vi "AdvancedConfig.vi"(8 "error in":errorcluster {"code" format="Error %.0f"}, 11 "MainFGV_data":T3={"TestDir"=path "", "TestName"="", "task"="", "data_file"=refnum, "AcqQueue"=refnum, "StartTime"=timestamp(0 s since 1904-01-01), "config_channels"=[], "DAQmx Device"="", "Advanced"={"rate"=1652.0, "duration"=1.0, "thr"=100.0, "preTrigger"=100.0, "cutoff"=-3.0, "Filtro"=enum."Desativado", "highPass"=1000.0, "lowPass"=1000.0, "updateTime"=50.0}, "running"=FALSE, "hammerIndex"=0, "session"="localhost"} {"Advanced"."updateTime" format="%#_g ms"; "Advanced"."lowPass" format="%#_g Hz"; "Advanced"."highPass" format="%#_g Hz"; "Advanced"."cutoff" format="%#_g dB"; "Advanced"."preTrigger" format="%#_g ms"; "Advanced"."thr" format="%#_g N"; "Advanced"."duration" format="%#_g s"; "Advanced"."rate" min=1652.0 max=51200.0 format="%#_g Hz"}) -> (0 "error out":errorcluster {"code" format="Error %.0f"}, 3 "MainFGV_data out":T3={"TestDir"=path "", "TestName"="", "task"="", "data_file"=refnum, "AcqQueue"=refnum, "StartTime"=timestamp(0 s since 1904-01-01), "config_channels"=[], "DAQmx Device"="", "Advanced"={"rate"=1652.0, "duration"=1.0, "thr"=100.0, "preTrigger"=100.0, "cutoff"=-3.0, "Filtro"=enum."Desativado", "highPass"=1000.0, "lowPass"=1000.0, "updateTime"=50.0}, "running"=FALSE, "hammerIndex"=0, "session"="localhost"} {"Advanced"."updateTime" format="%#_g ms"; "Advanced"."lowPass" format="%#_g Hz"; "Advanced"."highPass" format="%#_g Hz"; "Advanced"."cutoff" format="%#_g dB"; "Advanced"."preTrigger" format="%#_g ms"; "Advanced"."thr" format="%#_g N"; "Advanced"."duration" format="%#_g s"; "Advanced"."rate" min=1652.0 max=51200.0 format="%#_g Hz"})   [LabVIEW 2018]
uses:
  Processing/processing_mods.ctl
  MainFGV_data.ctl
  config_board.ctl
  AdvancedConfig.ctl
  NI9234_AcqRates.ctl
panel:
  in  "updateTime":dbl=50.0 caption="Intervalo de atualização" min=1.0 max=1000.0 format="%#_g ms"
  in  "rate":T1=enum."2048 Hz" caption="Taxa de aquisição"
  in  "lowPass":dbl=1000.0 caption="Passa baixa" format="%#_g Hz"
  in  "highPass":dbl=1.0 caption="Passa alta" format="%#_g Hz"
  in  "Filtro":T2(ring)=enum."Passa alta"
  in  "cutoff":dbl=-6.0 caption="Cutoff amplitude [dB]" max=-0.01 format="%#_g dB"
  in  "preTrigger":dbl=100.0 caption="Pre-trigger" min=0.0 max=60000.0 format="%#_g ms"
  in  "thr":dbl=10.0 caption="Limiar de força" min=1.0 format="%#_g N"
  in  "duration":dbl=1.0 caption="Duração" min=0.001 max=60.0 format="%#_g s"
  in  "cancel":bool
  in  "ok":bool
  # "Configurações avançadas"
  # "Detecção da batida"
  # "Apresentação do resultado"
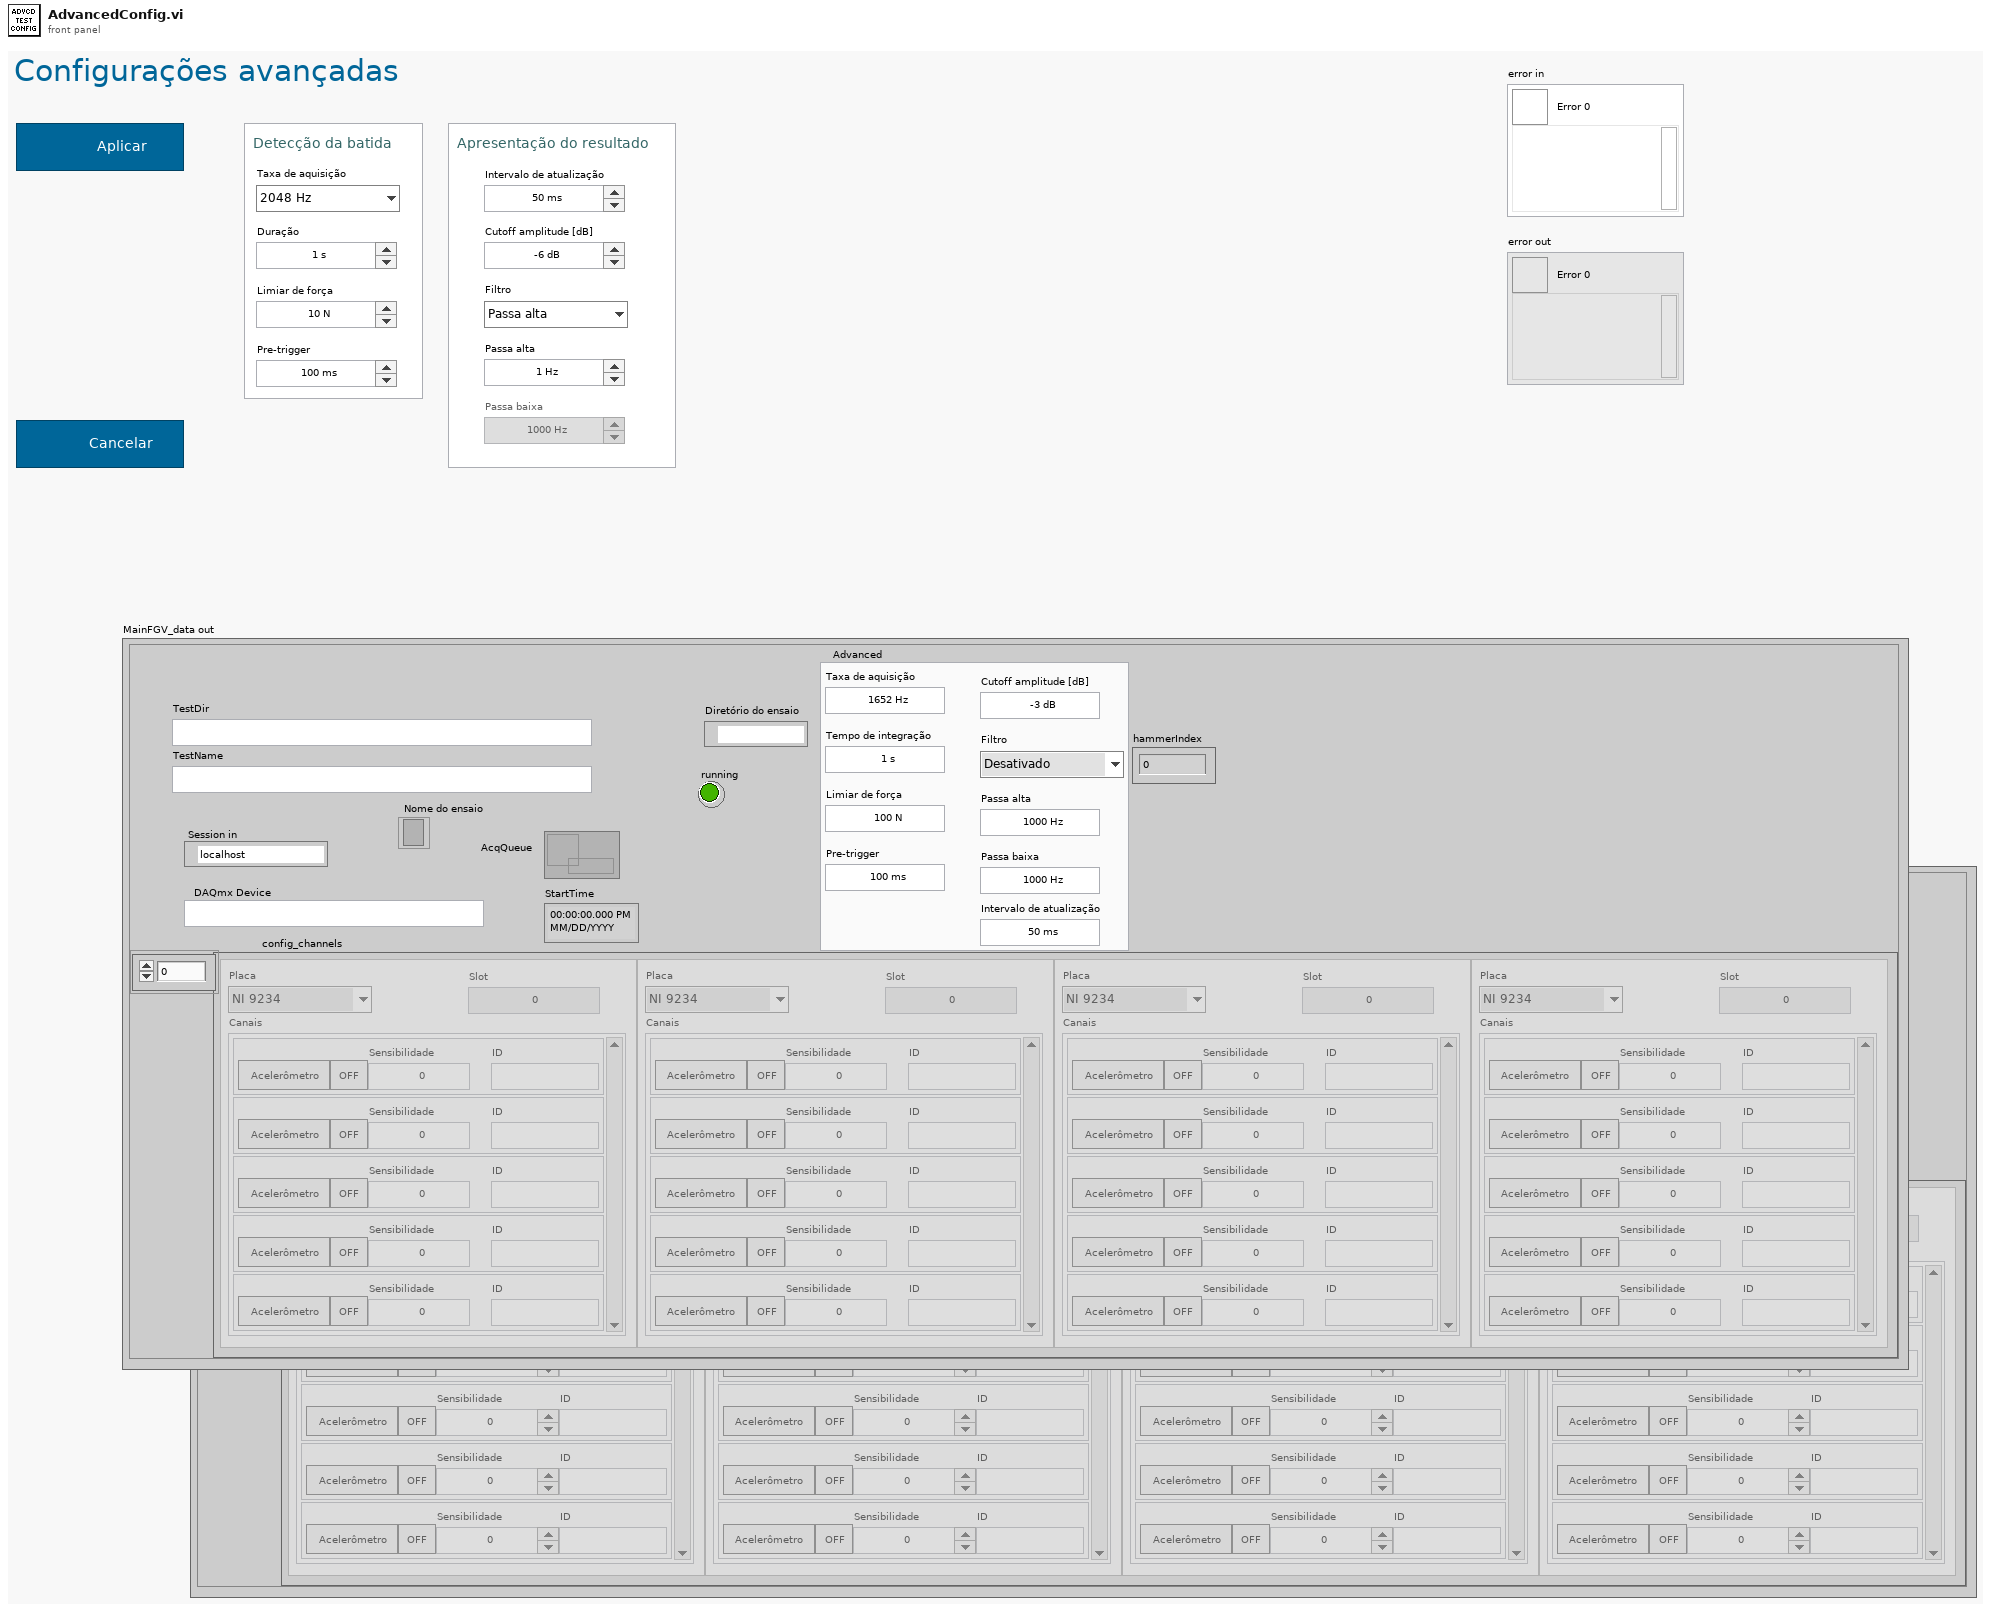
[diagram p1: front panel]
types:
  T1 = typedef "NI9234_AcqRates.ctl" = enum16{"51200 Hz", "25600 Hz", "17066 Hz", "12800 Hz", "10240 Hz", "8533 Hz", "7314 Hz", "6400 Hz", "5689 Hz", "5120 Hz", "4654 Hz", "4267 Hz", "3938 Hz", "3657 Hz", "3413 Hz", "3200 Hz", "3012 Hz", "2844 Hz", "2694 Hz", "2560 Hz", "2438 Hz", "2327 Hz", "2226 Hz", "2133 Hz", "2048 Hz", "1969 Hz", "1896 Hz", "1828 Hz", "1765 Hz", "1706 Hz", "1651 Hz"}
  T2 = enum16{"Desativado", "Passa banda", "Passa alta", "Passa baixa"}
  T3 = typedef "MainFGV_data.ctl" = cluster{"TestDir":path, "TestName":string, "task":refnum<k21>, "data_file":refnum<file>, "AcqQueue":refnum<queue>, "StartTime":timestamp, "config_channels":T4[], "DAQmx Device":tag, "Advanced":T5, "running":bool, "hammerIndex":i32, "session":refnum<k21>}
  T4 = typedef "config_board.ctl" = cluster{"board":enum16{"NI 9234", "NI 9205", "Não aplicável"}, "channels":cluster{"type":bool, "active":bool, "sens":dbl, "ID":string}[], "Slot":i32}
  T5 = typedef "AdvancedConfig.ctl" = cluster{"rate":dbl, "duration":dbl, "thr":dbl, "preTrigger":dbl, "cutoff":dbl, "Filtro":enum16{"Desativado", "Passa banda", "Passa alta", "Passa baixa"}, "highPass":dbl, "lowPass":dbl, "updateTime":dbl}
  T6 = typedef "processing_mods.ctl" = enum16{"newData", "SetConfig", "setHammer"}
  T7 = enum8{"Enabled", "Disabled", "Disabled and Grayed Out"}
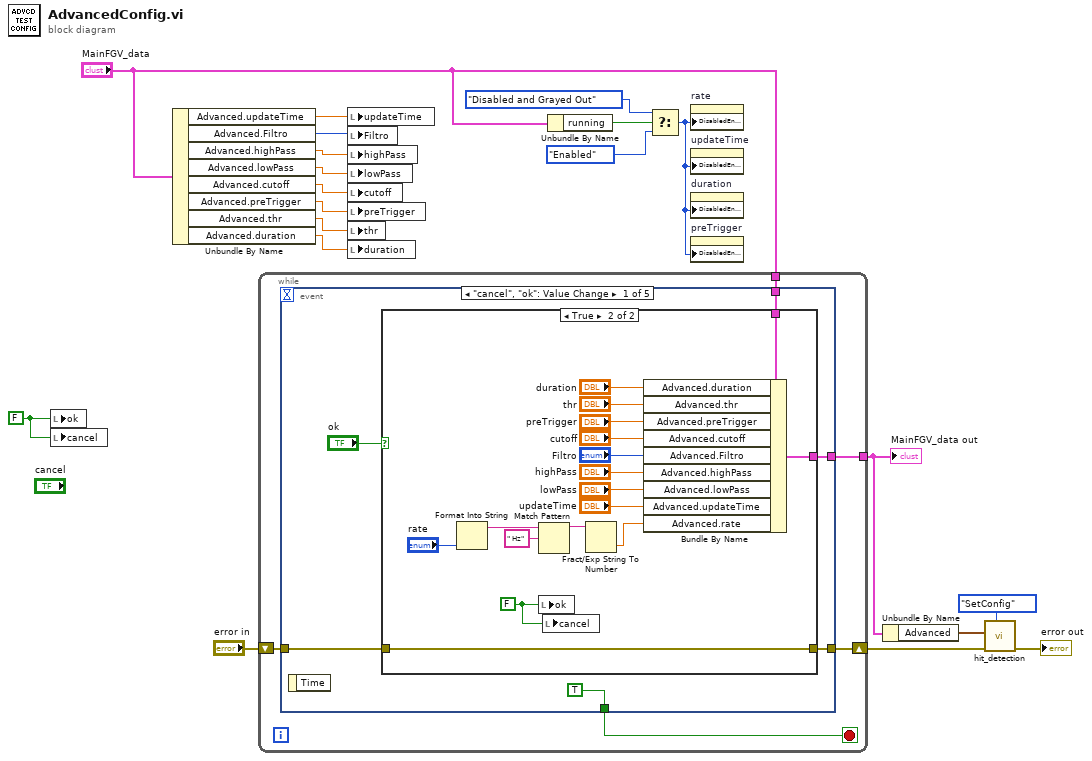
[diagram p0: block diagram]
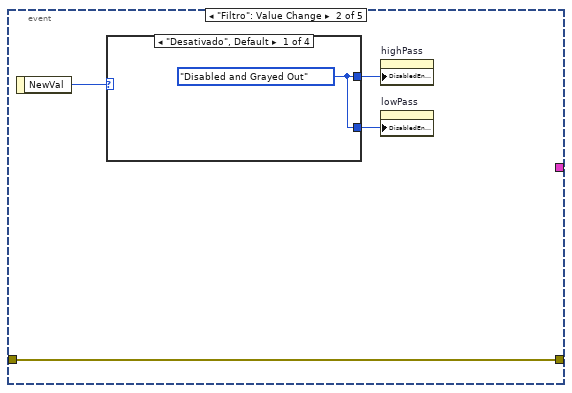
[diagram p3: hidden frame]
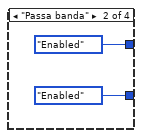
[diagram p4: hidden frame]
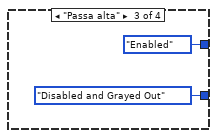
[diagram p5: hidden frame]
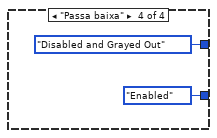
[diagram p6: hidden frame]
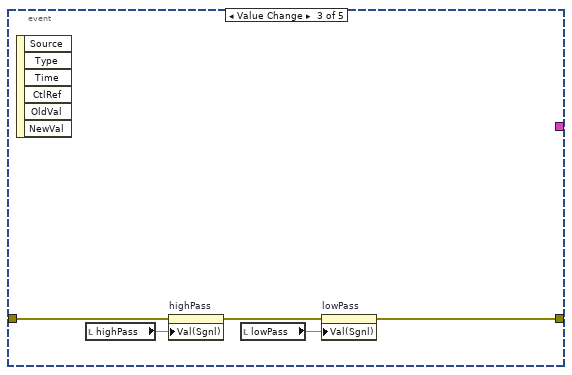
[diagram p7: hidden frame]
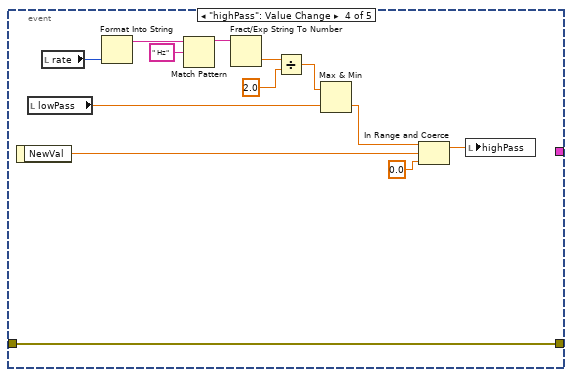
[diagram p8: hidden frame]
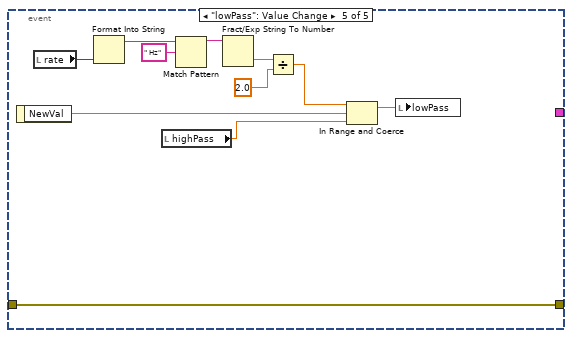
[diagram p9: hidden frame]
diagram:
  w19 = FALSE ("OK")
  n1 = local write "ok"(w19) -> ()
  n2 = local write "cancel"(w19) -> ()
  n3 = Unbundle By Name("MainFGV_data") -> ("Advanced.updateTime"=w8:dbl, "Advanced.Filtro"=w7:T2, "Advanced.highPass"=w6:dbl, "Advanced.lowPass"=w5:dbl, "Advanced.cutoff"=w4:dbl, "Advanced.preTrigger"=w3:dbl, "Advanced.thr"=w2:dbl, "Advanced.duration"=w1:dbl)
  n4 = while {
    shift-right: [w24] -> w14
    shift-left: "error in" -> [w21]
    tunnel: "MainFGV_data" -> [w23]
    tunnel: [w22] -> w13
    stop <- w25 stop-if-true
    n5 = event shown="[0] \"cancel\", \"ok\": Value Change" {
      selector: _ -> [_ _ _ _ _]
      dyn-events: _ -> [_ _ _ _ _]
      timeout: _ -> [_ _ _ _ _]
      tunnel: [TRUE ("OK") _ _ _ _] -> w25
      tunnel: w21 -> [w29 w51 w63 w67 w83]
      tunnel: [w28 w51 w62 w67 w83] -> w24
      tunnel: w23 -> [w31 _ _ _ _]
      tunnel: [w30 _ _ _ _] -> w22
      event "cancel", "ok": Value Change {
        n6 = event-data() -> ()  [unwired: 1 in, 1 out]
        n7 = case shown="True" "ok" {
          tunnel: w31 -> [w33 w50]
          tunnel: [w33 w49] -> w30
          tunnel: w29 -> [w32 w48]
          tunnel: [w32 w48] -> w28
          frame False {
          }
          frame True {
            w47 = FALSE ("OK")
            n8 = Format Into String("rate") -> (resulting string=w37:string)  [unwired: 3 in, 1 out]
            n9 = Match Pattern(string=w37, regular expression=" Hz") -> (before substring=w39:string)  [unwired: 1 in, 3 out]
            n10 = local write "ok"(w47) -> ()
            n11 = local write "cancel"(w47) -> ()
            n12 = Fract/Exp String To Number(string=w39) -> (number=w35:dbl)  [unwired: 3 in, 1 out]
            n13 = Bundle By Name(cluster=w50, "Advanced.duration"="duration", "Advanced.thr"="thr", "Advanced.preTrigger"="preTrigger", "Advanced.cutoff"="cutoff", "Advanced.Filtro"="Filtro", "Advanced.highPass"="highPass", "Advanced.lowPass"="lowPass", "Advanced.updateTime"="updateTime", "Advanced.rate"=w35) -> (w49:T3)
          }
        }
      }
      event "Filtro": Value Change {
        n14 = event-data() -> ("NewVal"=w54:T2)  [unwired: 1 in]
        n15 = case shown="\"Desativado\", Default" w54 {
          tunnel: [w55 T7."Enabled" ("Disabled") T7."Enabled" ("Disabled") T7."Disabled and Grayed Out" ("Disabled")] -> w53
          tunnel: [w55 T7."Enabled" ("Disabled") T7."Disabled and Grayed Out" ("Disabled") T7."Enabled" ("Disabled")] -> w52
          frame "Desativado", Default {
            w55 = T7."Disabled and Grayed Out" ("Disabled")
          }
          frame "Passa banda" {
          }
          frame "Passa alta" {
          }
          frame "Passa baixa" {
          }
        }
        n16 = property on="highPass" class="DigNum (strict)"("DisabledEnum"=w53) -> ()  [unwired: 2 in, 2 out]
        n17 = property on="lowPass" class="DigNum (strict)"("DisabledEnum"=w52) -> ()  [unwired: 2 in, 2 out]
      }
      event Value Change {
        n18 = event-data() -> ()  [unwired: 1 in, 6 out]
        n19 = local read "highPass"() -> (w66:dbl)
        n20 = property on="highPass" class="DigNum (strict)"(error in=w63, "Val(Sgnl)"=w66) -> (error out=w64:errorcluster)  [unwired: 1 in, 1 out]
        n21 = local read "lowPass"() -> (w65:dbl)
        n22 = property on="lowPass" class="DigNum (strict)"(error in=w64, "Val(Sgnl)"=w65) -> (error out=w62:errorcluster)  [unwired: 1 in, 1 out]
      }
      event "highPass": Value Change {
        n23 = event-data() -> ("NewVal"=w79:dbl)  [unwired: 1 in]
        n24 = local read "lowPass"() -> (w69:dbl)
        n25 = local read "rate"() -> (w76:T1)
        n26 = Format Into String(w76) -> (resulting string=w73:string)  [unwired: 3 in, 1 out]
        n27 = Match Pattern(string=w73, regular expression=" Hz") -> (before substring=w75:string)  [unwired: 1 in, 3 out]
        n28 = Fract/Exp String To Number(string=w75) -> (number=w72:dbl)  [unwired: 3 in, 1 out]
        n29 = Divide(x=w72, y=2.0) -> (x/y=w70:dbl)
        n30 = Max & Min(x=w70, y=w69) -> (min(x,y)=w68:dbl)  [unwired: 1 out]
        n31 = In Range and Coerce(upper limit=w68, x=w79, lower limit=0.0) -> (coerced(x)=w77:dbl)  [unwired: 1 out]
        n32 = local write "highPass"(w77) -> ()
      }
      event "lowPass": Value Change {
        n33 = event-data() -> ("NewVal"=w89:dbl)  [unwired: 1 in]
        n34 = local read "rate"() -> (w87:T1)
        n35 = Format Into String(w87) -> (resulting string=w84:string)  [unwired: 3 in, 1 out]
        n36 = local read "highPass"() -> (w88:dbl)
        n37 = Match Pattern(string=w84, regular expression=" Hz") -> (before substring=w86:string)  [unwired: 1 in, 3 out]
        n38 = Fract/Exp String To Number(string=w86) -> (number=w82:dbl)  [unwired: 3 in, 1 out]
        n39 = Divide(x=w82, y=2.0) -> (x/y=w81:dbl)
        n40 = In Range and Coerce(upper limit=w81, x=w89, lower limit=w88) -> (coerced(x)=w90:dbl)  [unwired: 1 out]
        n41 = local write "lowPass"(w90) -> ()
      }
    }
  }
  "MainFGV_data out" <- w13
  n42 = local write "updateTime"(w8) -> ()
  n43 = local write "Filtro"(w7) -> ()
  n44 = local write "highPass"(w6) -> ()
  n45 = local write "lowPass"(w5) -> ()
  n46 = local write "cutoff"(w4) -> ()
  n47 = local write "preTrigger"(w3) -> ()
  n48 = local write "thr"(w2) -> ()
  n49 = local write "duration"(w1) -> ()
  n50 = Unbundle By Name("MainFGV_data") -> ("running"=w18:bool)
  n51 = Select(t=T7."Disabled and Grayed Out" ("Disabled"), s=w18, f=T7."Enabled" ("Disabled")) -> (s? t:f=w15:T7)
  n52 = property on="rate" class="Enum (strict)"("DisabledEnum"=w15) -> ()  [unwired: 2 in, 2 out]
  n53 = property on="updateTime" class="DigNum (strict)"("DisabledEnum"=w15) -> ()  [unwired: 2 in, 2 out]
  n54 = property on="duration" class="DigNum (strict)"("DisabledEnum"=w15) -> ()  [unwired: 2 in, 2 out]
  n55 = property on="preTrigger" class="DigNum (strict)"("DisabledEnum"=w15) -> ()  [unwired: 2 in, 2 out]
  n56 = Unbundle By Name(w13) -> ("Advanced"=w10:T5)
  n57 = call "hit_detection.vi"("mod"=processing_mods."SetConfig", "error in"=w14, "config"=w10) -> ("error out"=→"error out":errorcluster)  [unwired: 8 in]
